vi "Global vars.vi"() -> ()   [LabVIEW 2014]
panel:
  out "charpos":u32
  in  "VRAMcolrs":string
  in  "VRAMchars":string
  in  "stop":bool
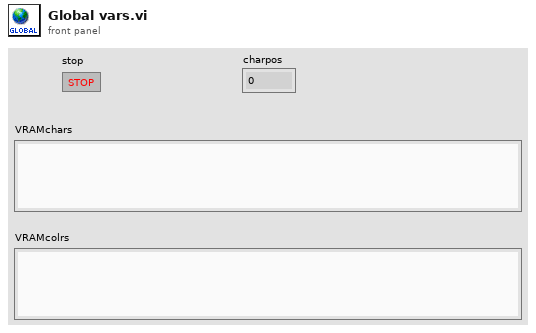
[diagram p1: front panel]
diagram:
